vi "1D_stats_labels.vi"(2 "Mode selector":T4(ring)=enum."4th Order Stats", 3 "Analysis Info Cluster":T1={"Colour"=0, "Inst type"=enum."Pitot-static tube", "Inst name"="Manometer voltage", "Symbol"="U", "Code name"="", "Extra Info"="U", "Inst Array"=enum."PWA", "Index"=0, "Voltage Index"=0, "Extra Titles"=[], "Extra Values"=[]}) -> (0 "Output":string[](array[string]))   [LabVIEW 2010]
uses:
  Controls/Analysis_info_cluster.ctl
  Controls/Inst_type.ctl
  Controls/Instrument_Array.ctl
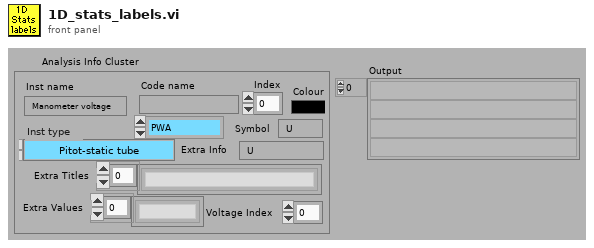
[diagram p1: front panel]
types:
  T1 = typedef "Analysis_info_cluster.ctl" = cluster{"Colour":u32, "Inst type":T2, "Inst name":string, "Symbol":string, "Code name":string, "Extra Info":string, "Inst Array":T3, "Index":i32, "Voltage Index":i32, "Extra Titles":string[], "Extra Values":string[]}
  T2 = typedef "Inst_type.ctl" = enum16{"Propeller anemometer", "Raw voltage", "Pressure Transducer", "Pitot-static tube", "Preston tube", "Hot wire", "Cross wire 1", "Cross wire 2", "Generic Linear", "Generic Polynomial", "Generic BackPoly", "Fast FID", "Thermocouple", "Cold wire", "Pulsed Wire", "LDA Vel", "LDA Tran time", "LDA Arr time"}
  T3 = typedef "Instrument_Array.ctl" = enum16{"PWA", "LDA", "Analogue"}
  T4 = enum16{"Mean only", "2nd Order Stats", "4th Order Stats"}
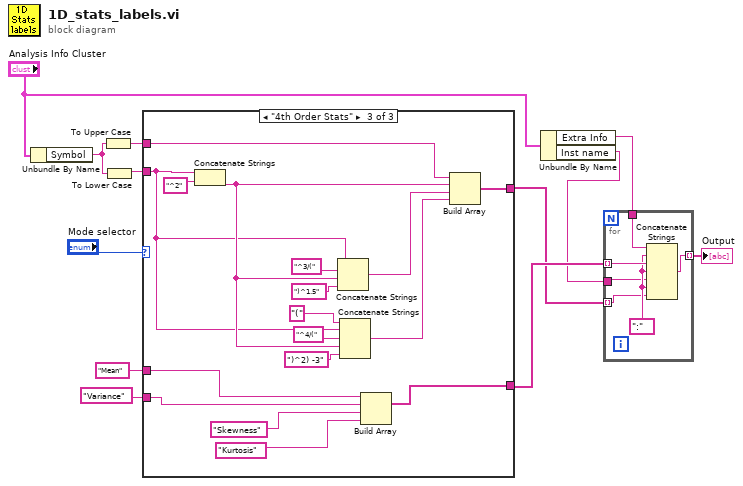
[diagram p0: block diagram]
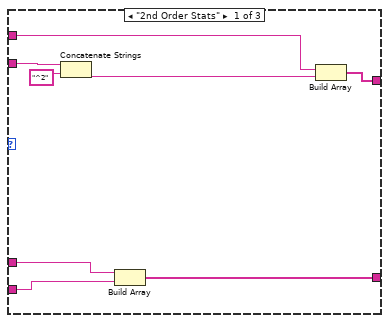
[diagram p2: hidden frame]
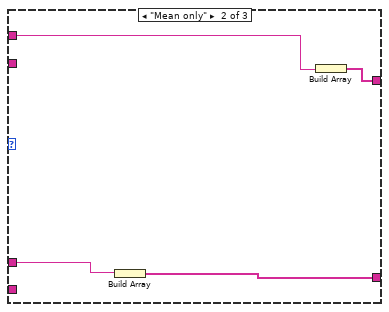
[diagram p3: hidden frame]
diagram:
  n1 = Unbundle By Name("Analysis Info Cluster") -> ("Symbol"=w6:string)
  n2 = To Upper Case(1:w6) -> (0:w11:string)
  n3 = To Lower Case(string=w6) -> (all lower case string=w10:string)
  n4 = case shown="\"4th Order Stats\"" "Mode selector" {
    tunnel: w11 -> [w20 w24 w41]
    tunnel: w10 -> [w17 _ w33]
    tunnel: [w18 w23 w31] -> w1
    tunnel: "Mean" -> [w15 w22 w27]
    tunnel: "Variance" -> [w14 _ w28]
    tunnel: [w13 w21 w26] -> w3
    frame "2nd Order Stats" {
      n5 = Concatenate Strings(w17, "^2") -> (w16:string)
      n6 = Build Array(w15, w14) -> (w13:string[])
      n7 = Build Array(w20, w16) -> (w18:string[])
    }
    frame "Mean only" {
      n8 = Build Array(w22) -> (w21:string[])
      n9 = Build Array(w24) -> (w23:string[])
    }
    frame "4th Order Stats" {
      n10 = Concatenate Strings(w33, "^2") -> (w34:string)
      n11 = Concatenate Strings(w33, "^3/(", w34, ")^1.5") -> (w37:string)
      n12 = Concatenate Strings("(", w33, "^4/(", w34, ")^2) -3") -> (w32:string)
      n13 = Build Array(w27, w28, "Skewness", "Kurtosis") -> (w26:string[])
      n14 = Build Array(w41, w34, w37, w32) -> (w31:string[])
    }
  }
  n15 = Unbundle By Name("Analysis Info Cluster") -> ("Extra Info"=w4:string, "Inst name"=w2:string)
  n16 = for {
    tunnel: [w47] -> w7 mode=indexing
    tunnel: w4 -> [w46]
    tunnel: w3 -> [w45] mode=indexing
    tunnel: w2 -> [w43]
    tunnel: w1 -> [w42] mode=indexing
    w44 = ":" ("Substring")
    n17 = Concatenate Strings(w46, w44, w45, w44, w43, w44, w42) -> (w47:string)
  }
  "Output" <- w7
